vi "SDSU_FindClk.vi"(6 "muxes":T2(array[cluster]), 9 "clk name":string, 10 "mux name":string, 11 "Table":string[][](table)) -> (0 "mux index":i32, 1 "found clk":bool, 2 "clk num":string, 3 "found mux":bool, 4 "muxes out":T1, 5 "mux num":string, 7 "board num":string)   [LabVIEW 2016]
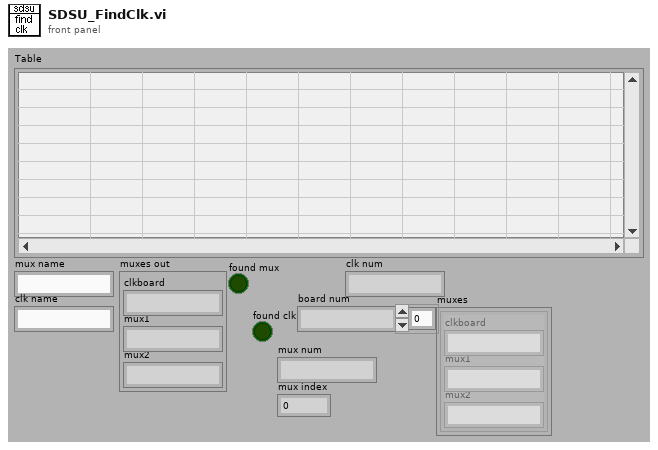
[diagram p1: front panel]
types:
  T1 = cluster{"clkboard":string, "mux1":string, "mux2":string}
  T2 = cluster{"clkboard":string, "mux1":string, "mux2":string}[]
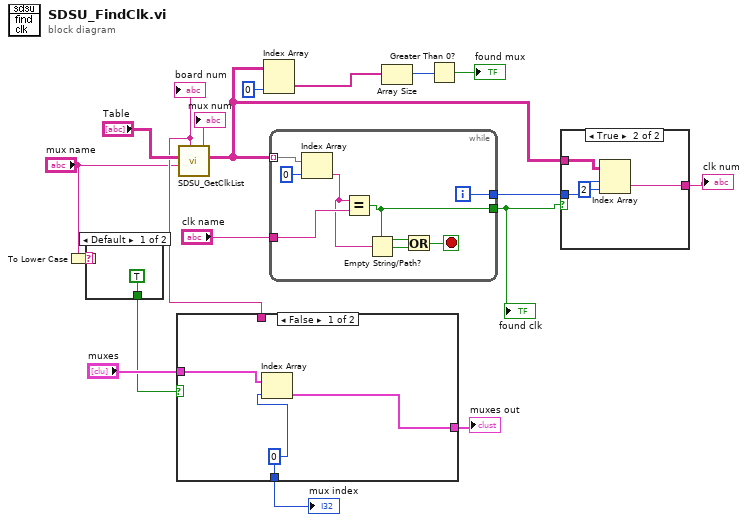
[diagram p0: block diagram]
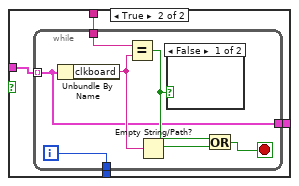
[diagram p2: hidden frame]
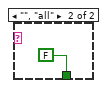
[diagram p4: hidden frame]
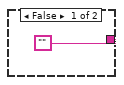
[diagram p5: hidden frame]
diagram:
  n1 = To Lower Case(string="mux name") -> (all lower case string=w2:string)
  n2 = case shown="Default" w2 {
    tunnel: [TRUE FALSE] -> w1
    frame Default {
    }
    frame "", "all" {
    }
  }
  n3 = call "SDSU_GetClkList.vi"("mux name"="mux name", "Table"="Table") -> ("cloks"=w13:string[][], "mux num"=→"mux num":string, "board num"=w6:string)  [unwired: 7 out]
  "board num" <- w6
  n4 = case shown="False" w1 {
    tunnel: "muxes" -> [w23 w27]
    tunnel: w6 -> [_ w26]
    tunnel: [w21 w25] -> w5
    tunnel: [w22 w24] -> w4
    frame False {
      w22 = 0
      n5 = Index Array(array=w23, index=w22) -> (element=w21:T1)
    }
    frame True {
      n6 = while {
        tunnel: w27 -> [w29] mode=indexing
        tunnel: w26 -> [w34]
        tunnel: [w29] -> w25
        tunnel: [w28] -> w24
        i -> [w28]
        stop <- w30 stop-if-true
        n7 = Unbundle By Name(w29) -> ("clkboard"=w32:string)
        n8 = Equal?(x=w34, y=w32) -> (x = y?=w33:bool)
        n9 = Empty String/Path?(string/path=w32) -> (empty?=w31:bool)
        n10 = case shown="False" w33 {
          frame False {
          }
          frame True {
          }
        }
        n11 = Or(x=w33, y=w31) -> (x .or. y?=w30:bool)
      }
    }
  }
  "muxes out" <- w5
  "mux index" <- w4
  n12 = Index Array(array=w13, index (col)=0 ("disabled index (col)")) -> (element=w11:string[])  [unwired: 1 in]
  n13 = while {
    tunnel: w13 -> [w42] mode=indexing
    tunnel: "clk name" -> [w40]
    tunnel: [w36] -> w16
    tunnel: [w35] -> w15
    i -> [w35]
    stop <- w37 stop-if-true
    n14 = Index Array(array=w42, index=0) -> (element=w39:string)
    n15 = Equal?(x=w39, y=w40) -> (x = y?=w36:bool)
    n16 = Empty String/Path?(string/path=w39) -> (empty?=w38:bool)
    n17 = Or(x=w36, y=w38) -> (x .or. y?=w37:bool)
  }
  "found clk" <- w16
  n18 = Array Size(array=w11) -> (size(s)=w10:i32)
  n19 = Greater Than 0?(x=w10) -> (x > 0?=→"found mux":bool)
  n20 = case shown="True" w16 {
    tunnel: w15 -> [_ w46]
    tunnel: w13 -> [_ w47]
    tunnel: ["" w44] -> w14
    frame False {
    }
    frame True {
      n21 = Index Array(array=w47, index (row)=w46, index (col)=2 ("disabled index (col)")) -> (element=w44:string)
    }
  }
  "clk num" <- w14
